vi "dht.vi"() -> ()   [LabVIEW 2020]
uses:
  <vilib>/Instr/_visa.llb/VISA Configure Serial Port (Instr).vi
  <vilib>/Analysis/Matrix/Numeric/Conversions/Array To Matrix - RA.vi
  <vilib>/Utility/file.llb/Write Delimited Spreadsheet (DBL).vi
  <vilib>/Analysis/Matrix/NI_Matrix.lvlib
panel:
  out "error out 6":errorcluster
  in  "append to file? (new file:F)":bool
  in  "file path (dialog if empty)":path
  in  "Tab Control":enum32{"Page 1", "Page 2", "Page 3"}(tab)
  out "Temp":dbl(slide) scale=0.0..100.0
  out "Humidity":dbl(slide) scale=0.0..100.0
  in  "temp point":u32(slide) scale=0.0..100.0
  in  "temp set":bool
  out "temp str":string
  in  "humid point 2":u32(slide) scale=0.0..100.0
  in  "humid set":bool
  out "humid str":string
  in  "fan set":bool
  in  "mist set":bool
  out "Waveform Chart":cluster{dbl, dbl}(graph)
  out "String 2":string="m00fe"
  out "String":string="f00fe"
  out "error out 5":errorcluster
  out "error out 4":errorcluster
  out "error out 3":errorcluster
  out "error out 2":errorcluster
  out "error out":errorcluster
  out "read buffer":string
  out "temp":dbl
  out "humid":dbl
  out "return count":u32
  in  "VISA resource name":refnum<visa-resource-name>
  in  "stop":bool
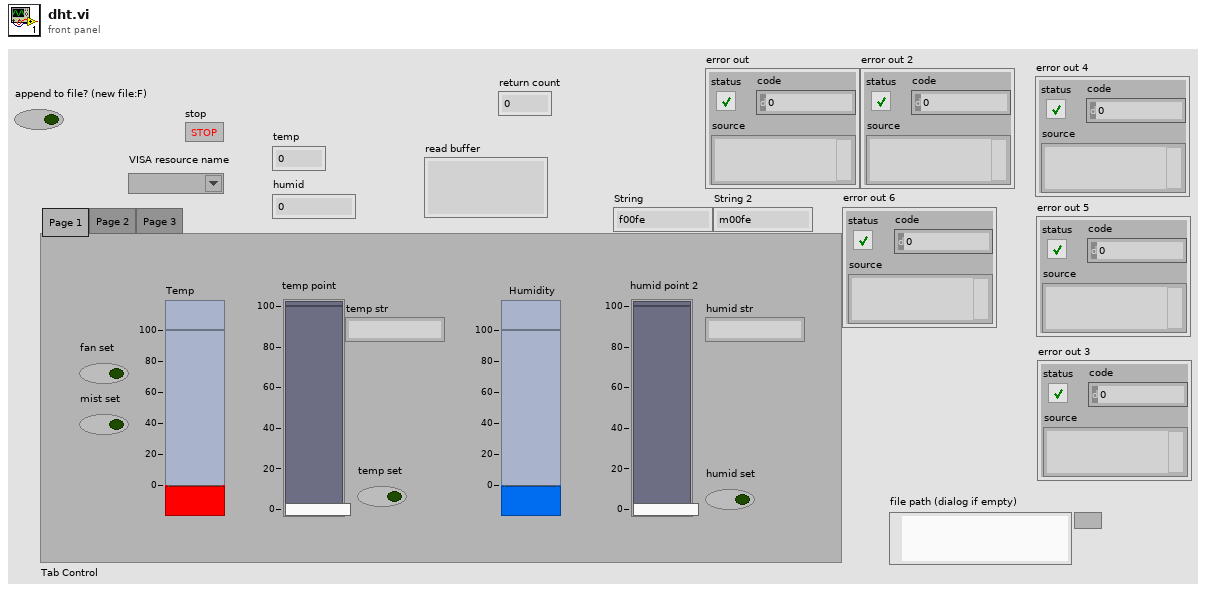
[diagram p1: front panel]
types:
  T1 = typedef "NI_Matrix.lvlib/RealMatrix.ctl" = dbl[][]
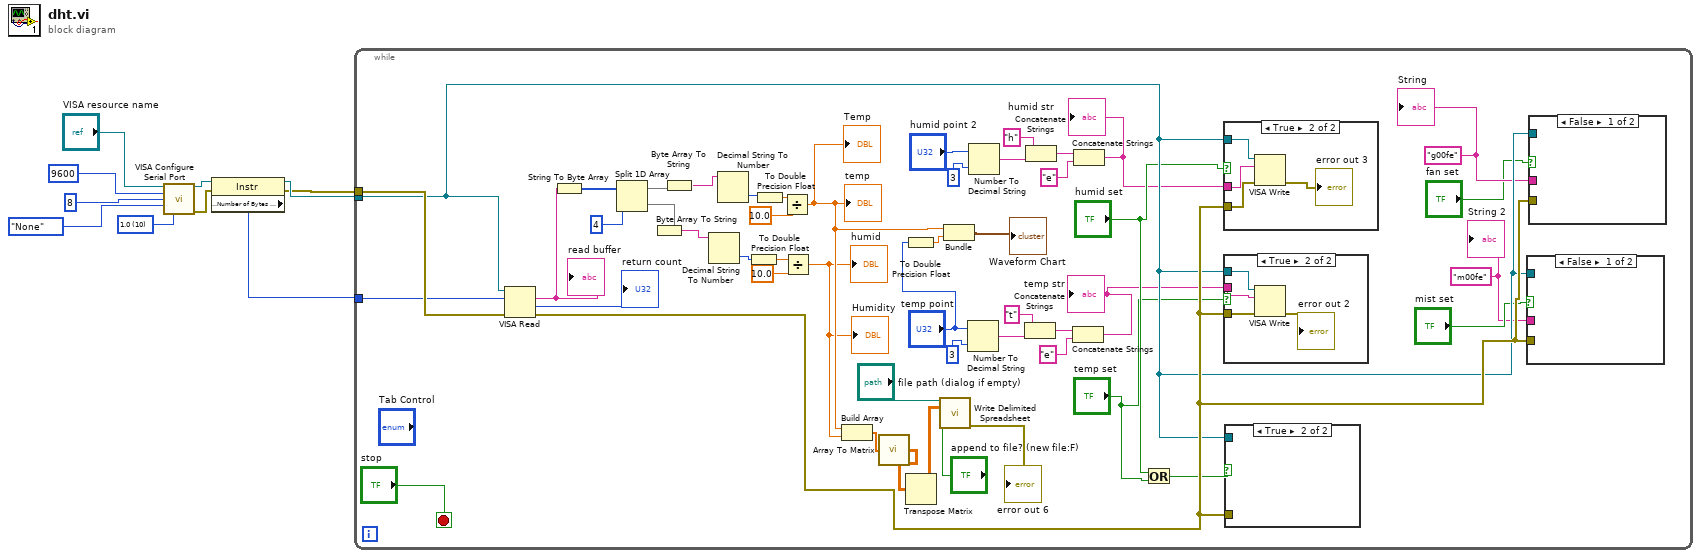
[diagram p0: block diagram]
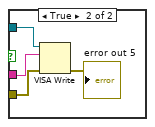
[diagram p2: hidden frame]
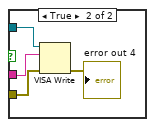
[diagram p3: hidden frame]
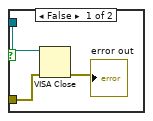
[diagram p6: hidden frame]
diagram:
  w6 = u16 10 items=["1.0"=10, "1.5"=15, "2.0"=20] ("stop bits (10: 1 bit)")
  n1 = call-poly "VISA Configure Serial Port"("VISA resource name"="VISA resource name", "baud rate (9600)"=u32 9600, "data bits (8)"=u16 8, "parity (0:none)"=enum16{"None", "Odd", "Even", "Mark", "Space"}."None", "stop bits (10: 1 bit)"=w6) -> ("VISA resource name out"=w5:refnum<visa-resource-name>, "error out"=w4:errorcluster)  [unwired: 9 in]
  n2 = property class="Instr"(reference=w5, error in=w4) -> (reference out=w3:refnum<visa-resource-name>, error out=w2:errorcluster, "Serial Settings:Number of Bytes at Serial Port"=w1:u32)
  n3 = while {
    tunnel: w3 -> [w56]
    tunnel: w2 -> [w59]
    tunnel: w1 -> [w58]
    stop <- "stop" stop-if-true
    w22 = "m00fe"
    w25 = "g00fe"
    n4 = VISA Read(VISA resource name=w56, byte count=w58, error in (no error)=w59) -> (read buffer=w42:string, return count=→"return count":u32, error out=w57:errorcluster)  [unwired: 1 out]
    "read buffer" <- w42
    n5 = String To Byte Array(string=w42) -> (unsigned byte array=w54:u8[])
    n6 = Split 1D Array(array=w54, index=4) -> (first subarray=w52:u8[], second subarray=w50:u8[])
    n7 = Byte Array To String(unsigned byte array=w50) -> (string=w51:string)
    n8 = Byte Array To String(unsigned byte array=w52) -> (string=w49:string)
    n9 = Decimal String To Number(string=w51) -> (number=w47:i32)  [unwired: 2 in, 1 out]
    n10 = Decimal String To Number(string=w49) -> (number=w48:i32)  [unwired: 2 in, 1 out]
    n11 = To Double Precision Float(number=w47) -> (double precision float=w44:dbl)
    n12 = To Double Precision Float(number=w48) -> (double precision float=w46:dbl)
    n13 = Divide(x=w46, y=10.0) -> (x/y=w17:dbl)
    "temp" <- w17
    "Temp" <- w17
    n14 = Divide(x=w44, y=10.0) -> (x/y=w16:dbl)
    "humid" <- w16
    "Humidity" <- w16
    n15 = Build Array(w17, w16) -> (w15:dbl[])
    n16 = call-poly <vilib>:"Array To Matrix.vi"("Real 1D Array"=w15) -> ("Real Matrix (Column Vector)"=w12:T1)
    n17 = To Double Precision Float(number="temp point") -> (double precision float=w20:dbl)
    n18 = Transpose Matrix(1:w12) -> (0:w11:T1)
    n19 = call-poly <vilib>:"Write Delimited Spreadsheet.vi"("file path (dialog if empty)"="file path (dialog if empty)", "2D data"=w11, "append to file? (new file:F)"="append to file? (new file:F)") -> ("error out"=→"error out 6":errorcluster)  [unwired: 11 in, 1 out]
    n20 = Bundle(w17, w20) -> (→"Waveform Chart":cluster{dbl, dbl})  [unwired: 1 in]
    n21 = Number To Decimal String(number="temp point", width (-)=i16 3) -> (decimal integer string=w36:string)
    n22 = Number To Decimal String(number="humid point 2", width (-)=i16 3) -> (decimal integer string=w39:string)
    n23 = Concatenate Strings("t" ("string"), w36) -> (w37:string)
    n24 = Concatenate Strings("h" ("string"), w39) -> (w40:string)
    n25 = Concatenate Strings(w37, "e" ("string")) -> (w27:string)
    "temp str" <- w27
    n26 = Concatenate Strings(w40, "e" ("string")) -> (w26:string)
    "humid str" <- w26
    n27 = Or(x="humid set", y="temp set") -> (x .or. y?=w41:bool)
    n28 = case shown="True" "humid set" {
      tunnel: w26 -> [_ w76]
      tunnel: w57 -> [_ w75]
      tunnel: w56 -> [_ w74]
      frame False {
      }
      frame True {
        n29 = VISA Write(VISA resource name=w74, write buffer=w76, error in (no error)=w75) -> (error out=→"error out 3":errorcluster)  [unwired: 2 out]
      }
    }
    n30 = case shown="True" "temp set" {
      tunnel: w27 -> [_ w72]
      tunnel: w57 -> [_ w71]
      tunnel: w56 -> [_ w70]
      frame False {
      }
      frame True {
        n31 = VISA Write(VISA resource name=w70, write buffer=w72, error in (no error)=w71) -> (error out=→"error out 2":errorcluster)  [unwired: 2 out]
      }
    }
    n32 = case shown="True" w41 {
      tunnel: w56 -> [w79 _]
      tunnel: w57 -> [w78 _]
      frame False {
        n33 = VISA Close(VISA resource name=w79, error in (no error)=w78) -> (error out=→"error out":errorcluster)
      }
      frame True {
      }
    }
    n34 = case shown="False" "mist set" {
      tunnel: w22 -> [_ w64]
      tunnel: w57 -> [_ w63]
      tunnel: w56 -> [_ w62]
      frame False {
      }
      frame True {
        n35 = VISA Write(VISA resource name=w62, write buffer=w64, error in (no error)=w63) -> (error out=→"error out 5":errorcluster)  [unwired: 2 out]
      }
    }
    n36 = case shown="False" "fan set" {
      tunnel: w25 -> [_ w68]
      tunnel: w57 -> [_ w67]
      tunnel: w56 -> [_ w66]
      frame False {
      }
      frame True {
        n37 = VISA Write(VISA resource name=w66, write buffer=w68, error in (no error)=w67) -> (error out=→"error out 4":errorcluster)  [unwired: 2 out]
      }
    }
    "String" <- w25
    "String 2" <- w22
  }
